vi "Microscope software version global.vi"() -> ()   [LabVIEW 2011]
panel:
  in  "Version String":string="Version 31  (3/15)"
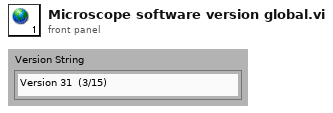
[diagram p1: front panel]
diagram:
